vi "runViWithFuncReturnOnly.vi"(8 "error in (no error)":errorcluster, 10 "vi path":path, 11 "SalProcess in":refnum<class "SalProcess.lvclass">) -> (0 "error out":errorcluster, 2 "function return":i32, 3 "SalProcess out":refnum<class "SalProcess.lvclass">)   [LabVIEW 2018, in "SalProcess.lvclass"]
doc: "Run the vi with the function return only."
uses:
  SalProcess.lvclass
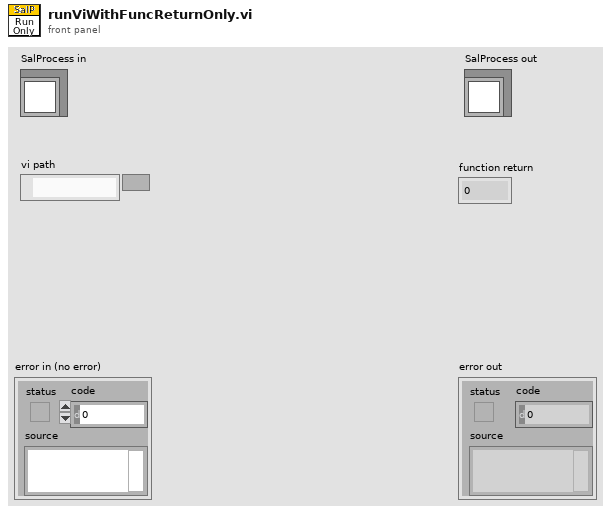
[diagram p1: front panel]
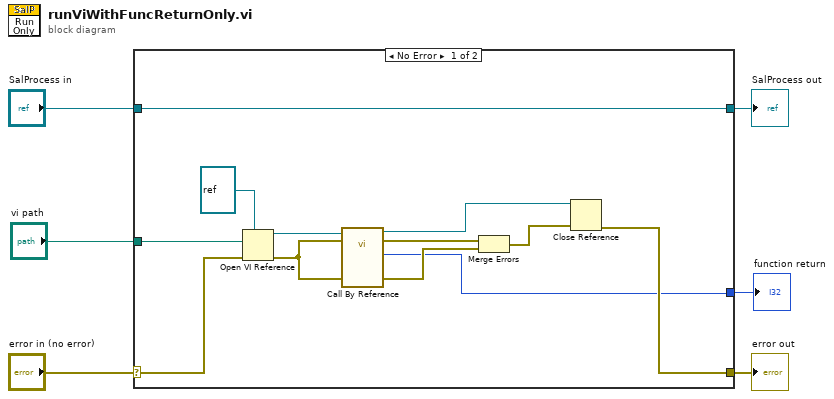
[diagram p0: block diagram]
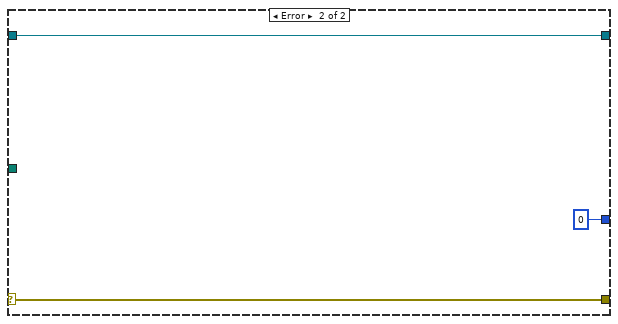
[diagram p2: hidden frame]
diagram:
  n1 = case shown="No Error" "error in (no error)" {
    selector: "error in (no error)" -> [w17 w21]
    tunnel: [w8 w21] -> w5
    tunnel: [w18 w20] -> w3
    tunnel: "SalProcess in" -> [w18 w20]
    tunnel: "vi path" -> [w16 _]
    tunnel: [w7 0 ("function return")] -> w1
    frame No Error {
      n2 = Open VI Reference(type specifier VI Refnum (for type only)=refnum<vi> refnum, vi path=w16, error in (no error)=w17) -> (vi reference=w14:refnum<vi>, error out=w13:errorcluster)  [unwired: 3 in]
      n3 = call-by-ref "?"(reference=w14, error in=w13, 8:"error in (no error)"=w13) -> (reference out=w10:refnum<vi>, error out=w12:errorcluster, 0:"error out"=w11:errorcluster, "function return"=w7:i32)  [unwired: 9 in]
      n4 = Merge Errors(w12, w11) -> (w9:errorcluster)
      n5 = Close Reference(reference=w10, error in (no error)=w9) -> (error out=w8:errorcluster)
    }
    frame Error {
    }
  }
  "error out" <- w5
  "SalProcess out" <- w3
  "function return" <- w1
